vi "insert message into map.vi"(8 "skip (F)":bool, 9 "message":T1 {"id" format="%x"; "data" format="%x"}, 11 "messages in":map{u32, T3}(c390)) -> (3 "messages out":map{u32, T3}(c390))   [LabVIEW 2024, in "atsj peakcan basic.lvlib"]
uses:
  atsj peakcan basic.lvlib
  message with stats.ctl
  message.ctl
  message type.ctl
  <vilib>/Utility/miscctls.llb/LVMapReplaceAction.ctl
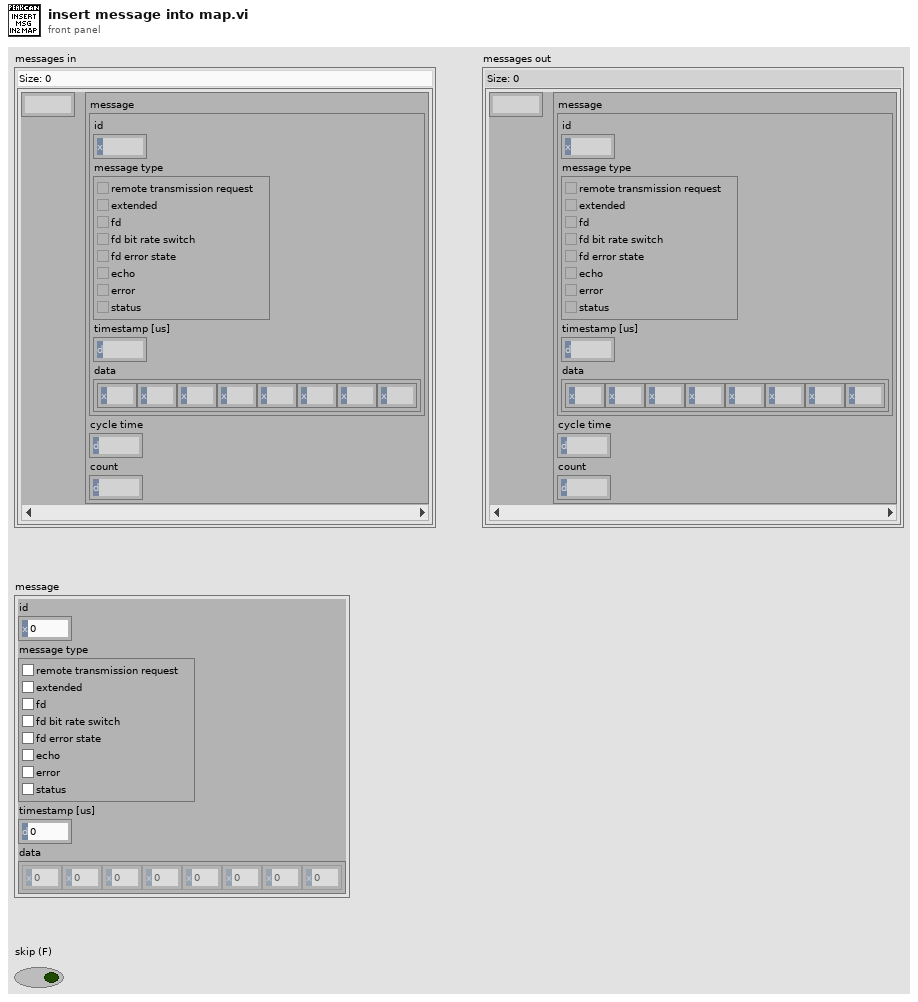
[diagram p1: front panel]
types:
  T1 = typedef "atsj peakcan basic.lvlib/message.ctl" = cluster{"id":u32, "message type":T2, "timestamp [us]":u64, "data":u8[]}
  T2 = typedef "atsj peakcan basic.lvlib/message type.ctl" = cluster{"remote transmission request ":bool, "extended":bool, "fd":bool, "fd bit rate switch":bool, "fd error state":bool, "echo":bool, "error":bool, "status":bool}
  T3 = typedef "atsj peakcan basic.lvlib/message with stats.ctl" = cluster{"message":T1, "cycle time":u64, "count":u64}
  T4 = typedef "LVMapReplaceAction.ctl" = enum32{"Modify Entry only if found", "Add or Modify Entry", "Delete Entry"}
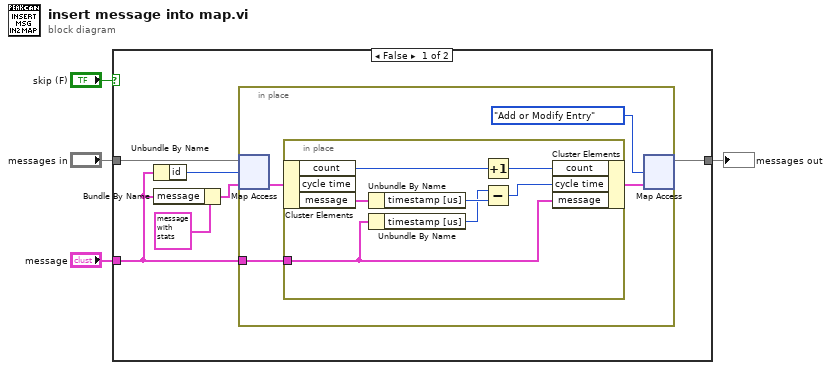
[diagram p0: block diagram]
diagram:
  n1 = case shown="False" "skip (F)" {
    tunnel: "message" -> [w8 _]
    tunnel: [w7 w22] -> w3
    tunnel: "messages in" -> [w10 w22]
    frame False {
      n2 = Unbundle By Name(w8) -> ("id"=w6:u32)
      n3 = Bundle By Name(cluster=T3 {"message"={"id"=0, "message type"={"remote transmission request "=FALSE, "extended"=FALSE, "fd"=FALSE, "fd bit rate switch"=FALSE, "fd error state"=FALSE, "echo"=FALSE, "error"=FALSE, "status"=FALSE}, "timestamp [us]"=0, "data"=[]}, "cycle time"=0, "count"=0}, "message"=w8) -> (w9:T3)
      n4 = in-place {
        in-place-border: w8 -> [w12]
        n5 = in-place-map #1(w10, w6, w9) -> (w14:T3)  [unwired: 1 out]
        n6 = in-place {
          in-place-border: w12 -> [w15]
          n7 = in-place-cluster #2(w14) -> ("count"=w20:u64, "message"=w21:T1)  [unwired: 1 out]
          n8 = Unbundle By Name(w21) -> ("timestamp [us]"=w18:u64)
          n9 = Unbundle By Name(w15) -> ("timestamp [us]"=w16:u64)
          n10 = Increment(x=w20) -> (x+1=w19:u64)
          n11 = Subtract(x=w16, y=w18) -> (x-y=w17:u64)
          n12 = in-place-cluster #2("count"=w19, "cycle time"=w17, "message"=w15) -> (w13:T3)
        }
        n13 = in-place-map #1(w13, LVMapReplaceAction."Add or Modify Entry" ("action")) -> (w7:map{u32, T3})  [unwired: 2 out]
      }
    }
    frame True {
    }
  }
  "messages out" <- w3
